vi "Read shutdown action config.vi"(8 "error in (no error)":errorcluster, 11 "Simple Sequencer TBM configuration in":refnum<class "Simple Sequencer TBM configuration.lvclass">) -> (0 "error out":errorcluster, 2 "shutdown action config":refnum<class "action configuration.lvclass">, 3 "Simple Sequencer TBM configuration out":refnum<class "Simple Sequencer TBM configuration.lvclass">)   [LabVIEW 2014, in "Simple Sequencer TBM configuration.lvclass"]
uses:
  Simple Sequencer TBM configuration.lvclass
  sequencer parent classes/action configuration parent/action configuration.lvclass
  Simple Sequencer TBM configuration.lvclass/Simple Sequencer TBM configuration.ctl
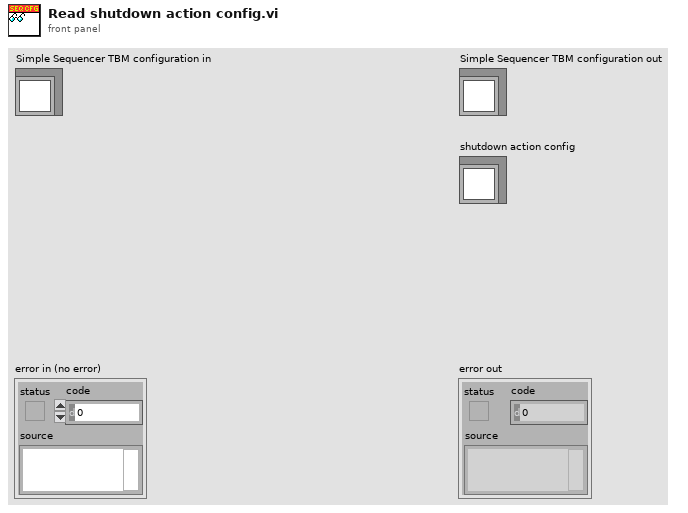
[diagram p1: front panel]
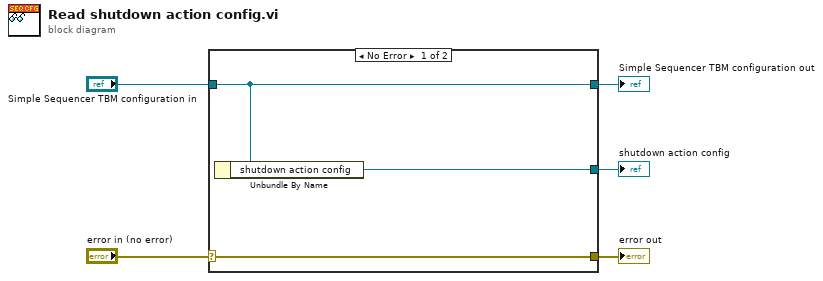
[diagram p0: block diagram]
diagram:
  n1 = case shown="No Error" "error in (no error)" {
    selector: "error in (no error)" -> [w8 w9]
    tunnel: [w8 w9] -> w4
    tunnel: [w7 w10] -> w2
    tunnel: "Simple Sequencer TBM configuration in" -> [w7 w10]
    tunnel: [w6 _] -> w1
    frame No Error {
      n2 = Unbundle By Name(w7) -> ("shutdown action config"=w6:refnum<class "action configuration.lvclass">)
    }
    frame Error {
    }
  }
  "error out" <- w4
  "Simple Sequencer TBM configuration out" <- w2
  "shutdown action config" <- w1
